vi "plain cycling.vi"() -> ()   [LabVIEW 2014]
doc: "This VI demonstrates the individual configuration of settings in I/W, W/I, and continuous operation modes.\n\nThis VI is not meant to be used with infusion-only models. \n\nNotes:\n(1) If continuous mode is selected, infuse volumes/rates will be used."
uses:
  <instrlib>/KD Scientific 2XX Series/KD Scientific 2XX Series.lvlib
panel:
  out "pressure mm Hg":dbl[](array[numeric])
  in  "Zero Error":dbl[](array[numeric])
  in  "Calibration factor":dbl[](array[numeric])
  out "Pressure mm Hg":dbl[](graph)
  out "Voltage from pressure transducer":dbl[](array[numeric])
  out "Data from Transducer":dynamicdata(graph) caption="Voltage from Transducer V"
  in  "stop (F)":bool
  in  "Number of Cycles":i32
  in  "Min Pressure":dbl
  in  "Max Pressure":dbl
  out "Units":string
  out "Delivered Volume":dbl
  in  "stop":bool
  out "Status":T1
  in  "Baud Rate (9600)":u32(ring)=9600 items=["300"=300, "1200"=1200, "2400"=2400, "4800"=4800, "9600"=9600]
  in  "Withdrawal Settings":T2={"Flow Rate (5)"=5.0, "Volume (10)"=10.0, "Volume Units (ml)"=enum."milliliters (ml)", "Rate Units (ml/min.)"=enum."milliliters per minute (ml/min.)"} {"Volume (10)" format="%#.3g"}
  in  "Diameter (8.75 mm)":dbl=8.75
  in  "Infusion Settings":T2={"Flow Rate (5)"=5.0, "Volume (10)"=10.0, "Volume Units (ml)"=enum."milliliters (ml)", "Rate Units (ml/min.)"=enum."milliliters per minute (ml/min.)"}
  in  "Address (0)":i32 format="%0.0f"
  in  "error in (no error)":errorcluster
  in  "VISA resource name":refnum<visa-resource-name>="COM1"
  # "RS-232 Settings"
  # "General Settings"
  # "Pump Status"
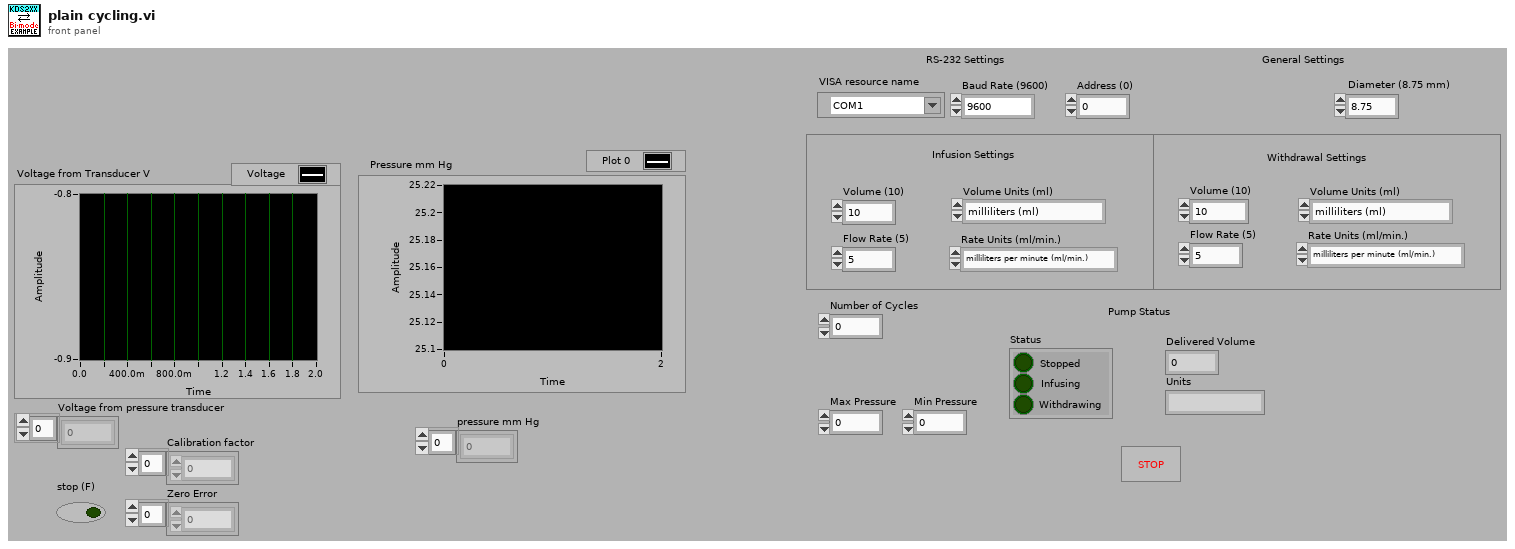
[diagram p1: front panel]
types:
  T1 = cluster{"Stopped":bool, "Infusing":bool, "Withdrawing":bool}
  T2 = cluster{"Flow Rate (5)":dbl, "Volume (10)":dbl, "Volume Units (ml)":enum16{"milliliters (ml)", "microliters (ul)"}, "Rate Units (ml/min.)":enum16{"milliliters per minute (ml/min.)", "milliliters per hour (ml/hr.)", "microliters per minute (ul/min.)", "microliters per hour (ul/hr.)"}}
  T3 = enum16{"milliliters per minute (ml/min.)", "milliliters per hour (ml/hr.)", "microliters per minute (ul/min.)", "microliters per hour (ul/hr.)"}
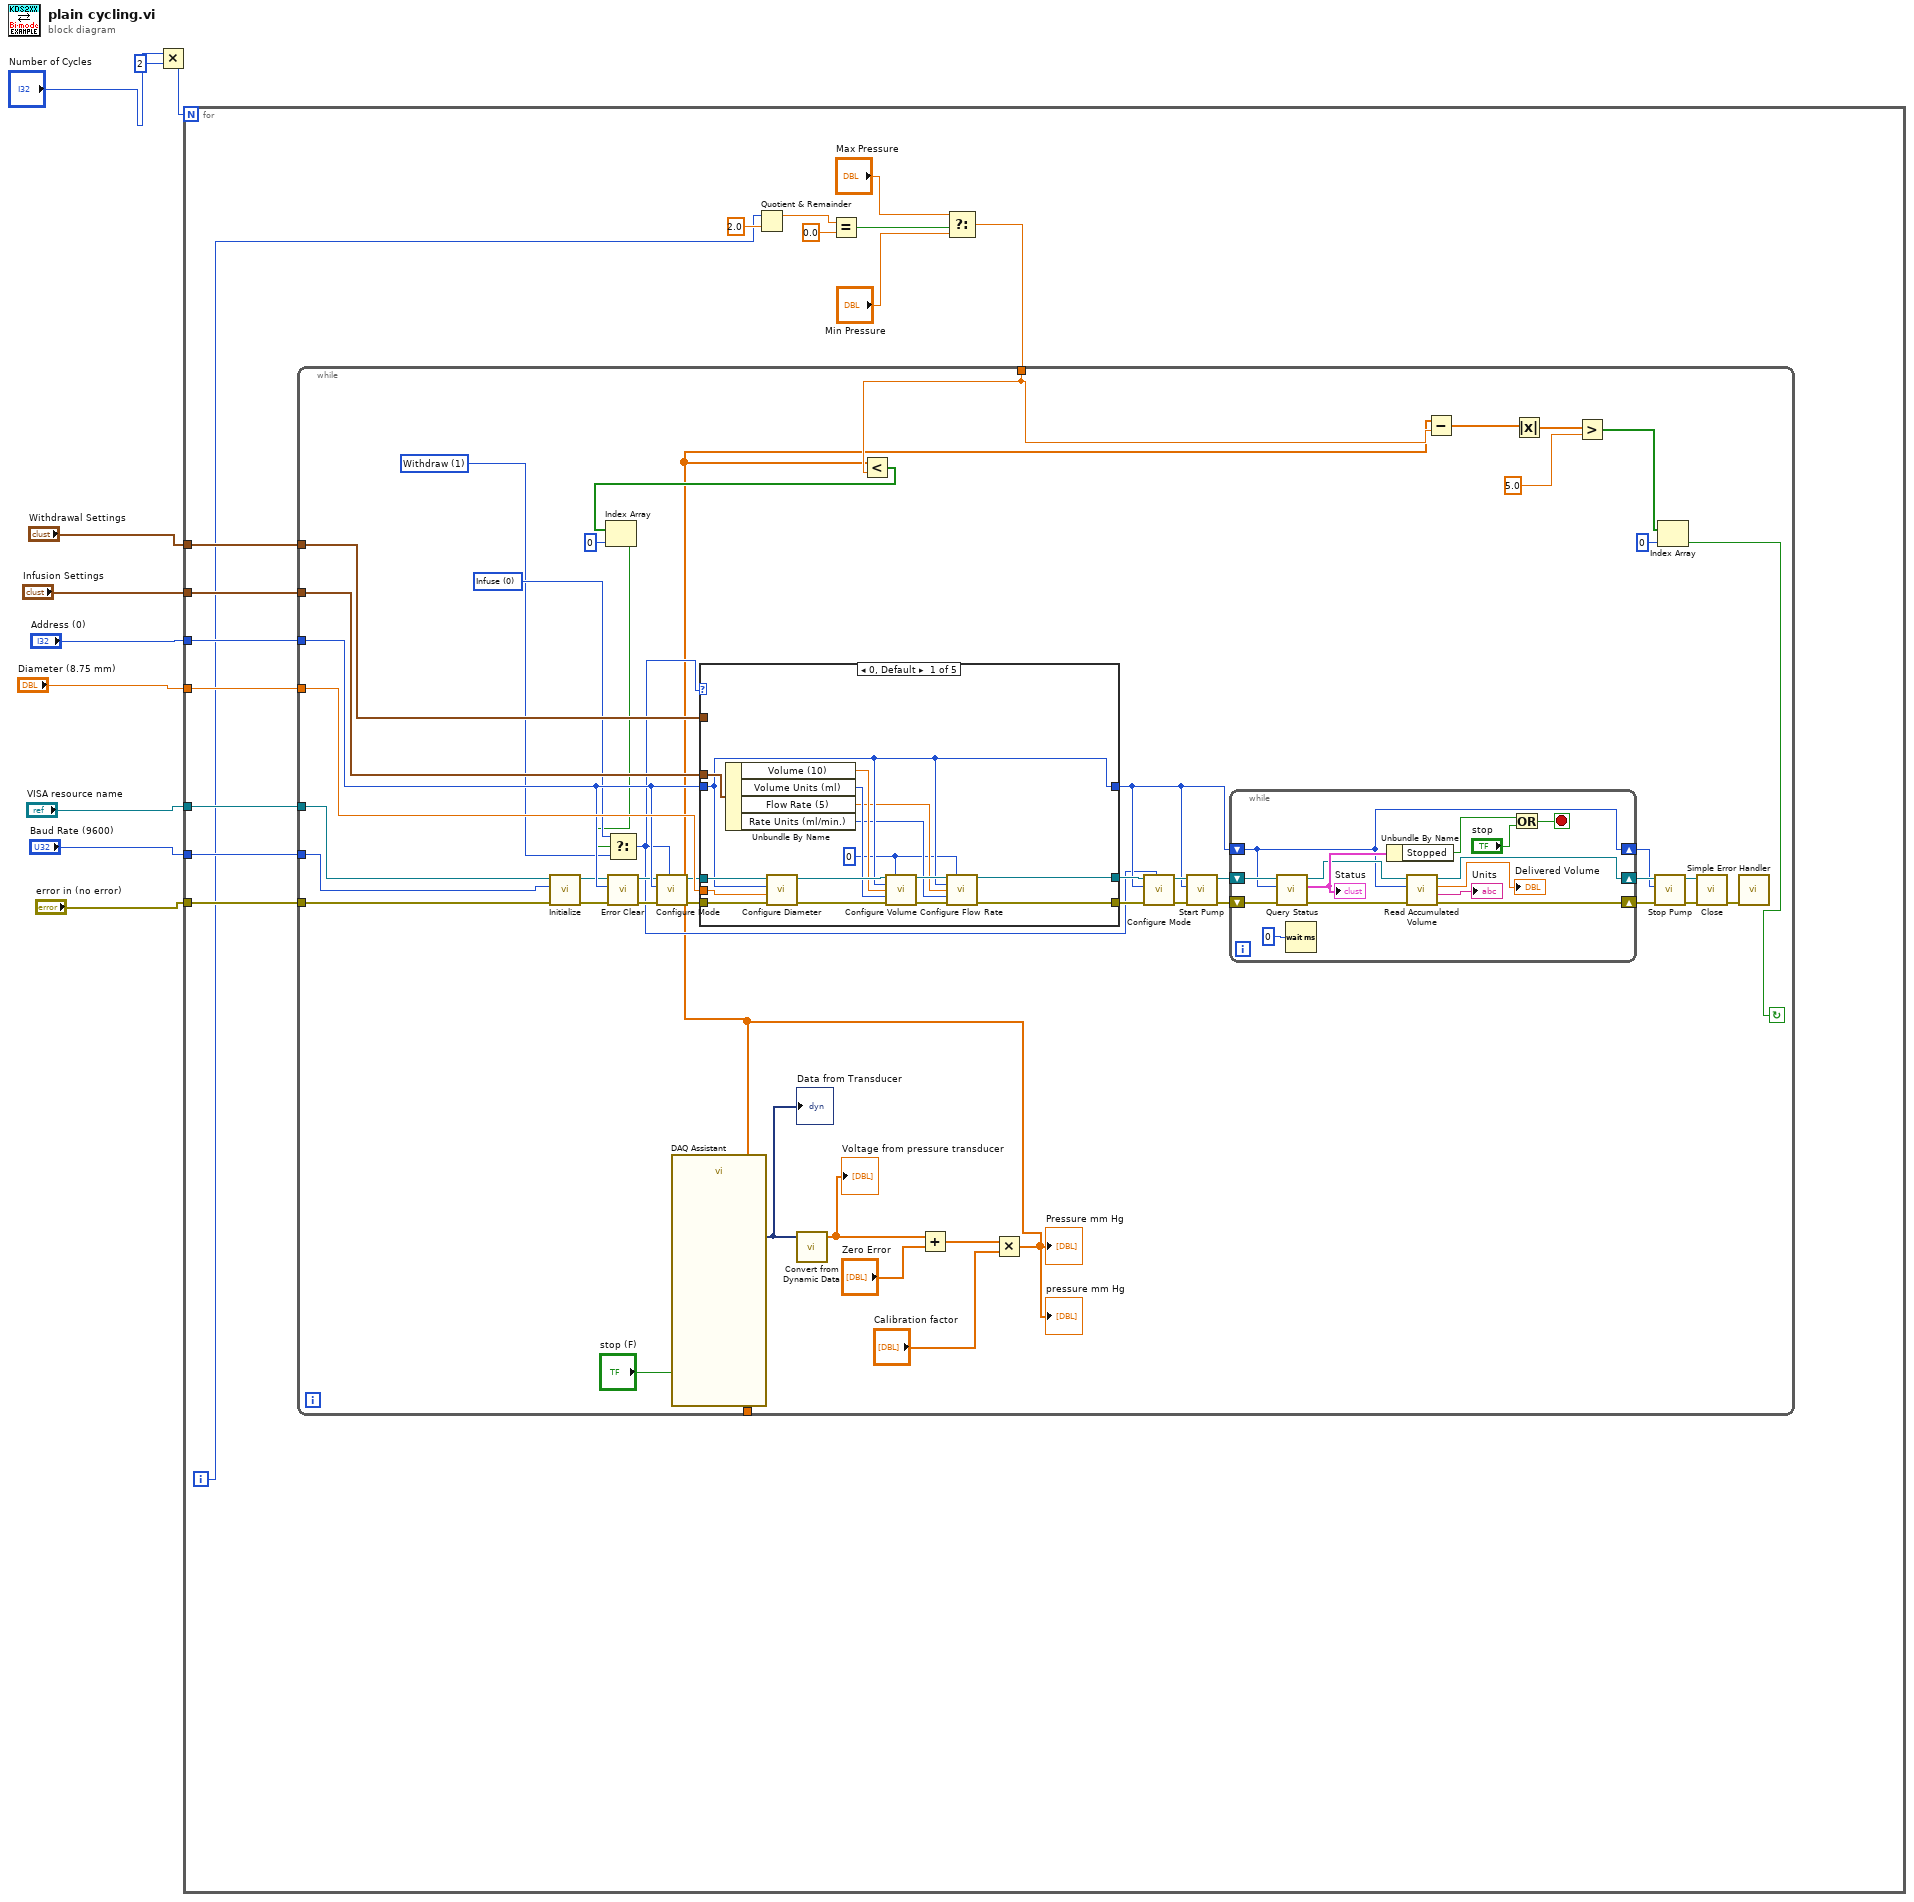
[diagram p0: block diagram]
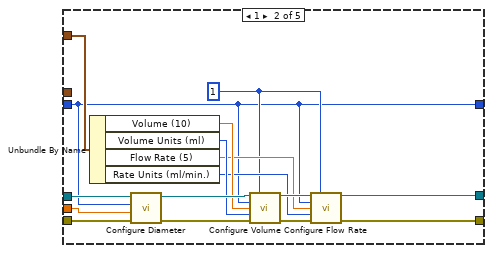
[diagram p2: hidden frame]
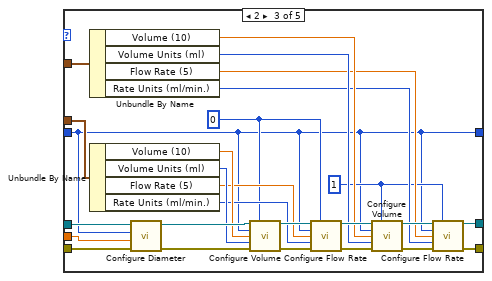
[diagram p3: hidden frame]
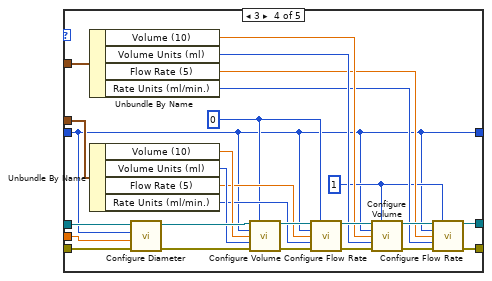
[diagram p4: hidden frame]
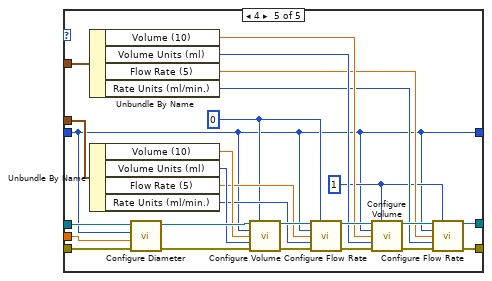
[diagram p5: hidden frame]
diagram:
  n1 = Multiply(x="Number of Cycles", y=2) -> (x*y=w1:i32)
  n2 = for {
    N: w1 -> [_]
    tunnel: "VISA resource name" -> [w25]
    tunnel: "error in (no error)" -> [w24]
    tunnel: "Infusion Settings" -> [w23]
    tunnel: "Withdrawal Settings" -> [w22]
    tunnel: "Diameter (8.75 mm)" -> [w21]
    tunnel: "Baud Rate (9600)" -> [w20]
    tunnel: "Address (0)" -> [w19]
    i -> [w17]
    n3 = Quotient & Remainder(x=w17, y=2.0) -> (x-y*floor(x/y)=w15:dbl)  [unwired: 1 out]
    n4 = Equal?(x=w15, y=0.0) -> (x = y?=w14:bool)
    n5 = Select(t="Max Pressure", s=w14, f="Min Pressure") -> (s? t:f=w11:dbl)
    n6 = while {
      tunnel: w25 -> [w71]
      tunnel: w24 -> [w70]
      tunnel: w23 -> [w69]
      tunnel: w22 -> [w68]
      tunnel: w21 -> [w67]
      tunnel: w20 -> [w66]
      tunnel: w19 -> [w65]
      tunnel: w11 -> [w42]
      tunnel: [w26] -> _
      stop <- w33 continue-if-true
      w44 = u16 1 items=["Withdraw"=1]
      w45 = u16 0 items=["Infuse"] ("Mode (infuse)")
      n7 = call <instrlib>:"Initialize.vi"("error in (no error)"=w70, "Baud Rate (9600)"=w66, "VISA resource name"=w71) -> ("error out"=w47:errorcluster, "VISA resource name out"=w46:refnum<visa-resource-name>)  [unwired: 7 in]
      n8 = call <instrlib>:"Error Clear.vi"("error in (no error)"=w47, "Address (0)"=w65, "VISA resource name"=w46) -> ("error out"=w48:errorcluster, "VISA resource name out"=w49:refnum<visa-resource-name>)  [unwired: 6 in, 1 out]
      n9 = call "DAQ Assistant"("stop (F)"="stop (F)") -> ("data"=w32:dynamicdata)  [unwired: 15 in, 3 out]
      "Data from Transducer" <- w32
      n10 = call "Convert from Dynamic Data"("Dynamic Data Type"=w32) -> ("Array"=w29:dbl[])  [unwired: 3 in]
      "Voltage from pressure transducer" <- w29
      n11 = Add(x=w29, y="Zero Error") -> (x+y=w31:dbl[])
      n12 = Multiply(x=w31, y="Calibration factor") -> (x*y=w26:dbl[])
      "Pressure mm Hg" <- w26
      "pressure mm Hg" <- w26
      n13 = Less?(x=w26, y=w42) -> (x < y?=w38:bool[])
      n14 = Index Array(array=w38, index=0) -> (element=w36:bool)
      n15 = Select(t=w45, s=w36, f=w44) -> (s? t:f=w43:u16)
      n16 = call <instrlib>:"Configure Mode.vi"("Mode (infuse)"=w43, "error in (no error)"=w48, "Address (0)"=w65, "VISA resource name"=w49) -> ("error out"=w51:errorcluster, "VISA resource name out"=w50:refnum<visa-resource-name>)  [unwired: 6 in]
      n17 = case shown="0, Default" w43 {
        tunnel: w69 -> [w81 _ w129 w155 w181]
        tunnel: w68 -> [_ w103 w128 w154 w180]
        tunnel: w50 -> [w87 w102 w127 w153 w179]
        tunnel: w51 -> [w86 w98 w126 w152 w178]
        tunnel: w67 -> [w80 w94 w109 w135 w161]
        tunnel: [w79 w88 w104 w130 w156] -> w52
        tunnel: w65 -> [w79 w88 w104 w130 w156]
        tunnel: [w74 w99 w106 w132 w158] -> w56
        tunnel: [w73 w95 w105 w131 w157] -> w55
        frame 0, Default {
          w72 = 0
          n18 = Unbundle By Name(w81) -> ("Volume (10)"=w78:dbl, "Volume Units (ml)"=w77:enum16{"milliliters (ml)", "microliters (ul)"}, "Flow Rate (5)"=w76:dbl, "Rate Units (ml/min.)"=w75:T3)
          n19 = call <instrlib>:"Configure Diameter.vi"("error in (no error)"=w86, "Diameter (8.75 mm)"=w80, "Address (0)"=w79, "VISA resource name"=w87) -> ("error out"=w84:errorcluster, "VISA resource name out"=w85:refnum<visa-resource-name>)  [unwired: 6 in]
          n20 = call <instrlib>:"Configure Volume.vi"("VISA resource name"=w85, "Mode (infuse)"=w72, "Address (0)"=w79, "Volume (100)"=w78, "Units (0: milliliters)"=w77, "error in (no error)"=w84) -> ("VISA resource name out"=w83:refnum<visa-resource-name>, "error out"=w82:errorcluster)  [unwired: 8 in]
          n21 = call <instrlib>:"Configure Flow Rate.vi"("VISA resource name"=w83, "Mode (infuse)"=w72, "Address (0)"=w79, "Flow Rate (5)"=w76, "Units (0: milliliters per minute)"=w75, "error in (no error)"=w82) -> ("VISA resource name out"=w74:refnum<visa-resource-name>, "error out"=w73:errorcluster)  [unwired: 8 in]
        }
        frame 1 {
          w89 = 1
          n22 = Unbundle By Name(w103) -> ("Volume (10)"=w93:dbl, "Volume Units (ml)"=w92:enum16{"milliliters (ml)", "microliters (ul)"}, "Flow Rate (5)"=w91:dbl, "Rate Units (ml/min.)"=w90:T3)
          n23 = call <instrlib>:"Configure Diameter.vi"("error in (no error)"=w98, "Diameter (8.75 mm)"=w94, "Address (0)"=w88, "VISA resource name"=w102) -> ("error out"=w97:errorcluster, "VISA resource name out"=w101:refnum<visa-resource-name>)  [unwired: 6 in]
          n24 = call <instrlib>:"Configure Volume.vi"("VISA resource name"=w101, "Mode (infuse)"=w89, "Address (0)"=w88, "Volume (100)"=w93, "Units (0: milliliters)"=w92, "error in (no error)"=w97) -> ("VISA resource name out"=w100:refnum<visa-resource-name>, "error out"=w96:errorcluster)  [unwired: 8 in]
          n25 = call <instrlib>:"Configure Flow Rate.vi"("VISA resource name"=w100, "Mode (infuse)"=w89, "Address (0)"=w88, "Flow Rate (5)"=w91, "Units (0: milliliters per minute)"=w90, "error in (no error)"=w96) -> ("VISA resource name out"=w99:refnum<visa-resource-name>, "error out"=w95:errorcluster)  [unwired: 8 in]
        }
        frame 2 {
          w107 = 1
          w108 = 0
          n26 = Unbundle By Name(w128) -> ("Volume (10)"=w113:dbl, "Volume Units (ml)"=w112:enum16{"milliliters (ml)", "microliters (ul)"}, "Flow Rate (5)"=w111:dbl, "Rate Units (ml/min.)"=w110:T3)
          n27 = Unbundle By Name(w129) -> ("Volume (10)"=w117:dbl, "Volume Units (ml)"=w116:enum16{"milliliters (ml)", "microliters (ul)"}, "Flow Rate (5)"=w115:dbl, "Rate Units (ml/min.)"=w114:T3)
          n28 = call <instrlib>:"Configure Diameter.vi"("error in (no error)"=w126, "Diameter (8.75 mm)"=w109, "Address (0)"=w104, "VISA resource name"=w127) -> ("error out"=w121:errorcluster, "VISA resource name out"=w125:refnum<visa-resource-name>)  [unwired: 6 in]
          n29 = call <instrlib>:"Configure Volume.vi"("VISA resource name"=w125, "Mode (infuse)"=w108, "Address (0)"=w104, "Volume (100)"=w117, "Units (0: milliliters)"=w116, "error in (no error)"=w121) -> ("VISA resource name out"=w124:refnum<visa-resource-name>, "error out"=w120:errorcluster)  [unwired: 8 in]
          n30 = call <instrlib>:"Configure Flow Rate.vi"("VISA resource name"=w124, "Mode (infuse)"=w108, "Address (0)"=w104, "Flow Rate (5)"=w115, "Units (0: milliliters per minute)"=w114, "error in (no error)"=w120) -> ("VISA resource name out"=w123:refnum<visa-resource-name>, "error out"=w119:errorcluster)  [unwired: 8 in]
          n31 = call <instrlib>:"Configure Volume.vi"("VISA resource name"=w123, "Mode (infuse)"=w107, "Address (0)"=w104, "Volume (100)"=w113, "Units (0: milliliters)"=w112, "error in (no error)"=w119) -> ("VISA resource name out"=w122:refnum<visa-resource-name>, "error out"=w118:errorcluster)  [unwired: 8 in]
          n32 = call <instrlib>:"Configure Flow Rate.vi"("VISA resource name"=w122, "Mode (infuse)"=w107, "Address (0)"=w104, "Flow Rate (5)"=w111, "Units (0: milliliters per minute)"=w110, "error in (no error)"=w118) -> ("VISA resource name out"=w106:refnum<visa-resource-name>, "error out"=w105:errorcluster)  [unwired: 8 in]
        }
        frame 3 {
          w133 = 1
          w134 = 0
          n33 = Unbundle By Name(w154) -> ("Volume (10)"=w139:dbl, "Volume Units (ml)"=w138:enum16{"milliliters (ml)", "microliters (ul)"}, "Flow Rate (5)"=w137:dbl, "Rate Units (ml/min.)"=w136:T3)
          n34 = Unbundle By Name(w155) -> ("Volume (10)"=w143:dbl, "Volume Units (ml)"=w142:enum16{"milliliters (ml)", "microliters (ul)"}, "Flow Rate (5)"=w141:dbl, "Rate Units (ml/min.)"=w140:T3)
          n35 = call <instrlib>:"Configure Diameter.vi"("error in (no error)"=w152, "Diameter (8.75 mm)"=w135, "Address (0)"=w130, "VISA resource name"=w153) -> ("error out"=w147:errorcluster, "VISA resource name out"=w151:refnum<visa-resource-name>)  [unwired: 6 in]
          n36 = call <instrlib>:"Configure Volume.vi"("VISA resource name"=w151, "Mode (infuse)"=w134, "Address (0)"=w130, "Volume (100)"=w143, "Units (0: milliliters)"=w142, "error in (no error)"=w147) -> ("VISA resource name out"=w150:refnum<visa-resource-name>, "error out"=w146:errorcluster)  [unwired: 8 in]
          n37 = call <instrlib>:"Configure Flow Rate.vi"("VISA resource name"=w150, "Mode (infuse)"=w134, "Address (0)"=w130, "Flow Rate (5)"=w141, "Units (0: milliliters per minute)"=w140, "error in (no error)"=w146) -> ("VISA resource name out"=w149:refnum<visa-resource-name>, "error out"=w145:errorcluster)  [unwired: 8 in]
          n38 = call <instrlib>:"Configure Volume.vi"("VISA resource name"=w149, "Mode (infuse)"=w133, "Address (0)"=w130, "Volume (100)"=w139, "Units (0: milliliters)"=w138, "error in (no error)"=w145) -> ("VISA resource name out"=w148:refnum<visa-resource-name>, "error out"=w144:errorcluster)  [unwired: 8 in]
          n39 = call <instrlib>:"Configure Flow Rate.vi"("VISA resource name"=w148, "Mode (infuse)"=w133, "Address (0)"=w130, "Flow Rate (5)"=w137, "Units (0: milliliters per minute)"=w136, "error in (no error)"=w144) -> ("VISA resource name out"=w132:refnum<visa-resource-name>, "error out"=w131:errorcluster)  [unwired: 8 in]
        }
        frame 4 {
          w159 = 1
          w160 = 0
          n40 = Unbundle By Name(w180) -> ("Volume (10)"=w165:dbl, "Volume Units (ml)"=w164:enum16{"milliliters (ml)", "microliters (ul)"}, "Flow Rate (5)"=w163:dbl, "Rate Units (ml/min.)"=w162:T3)
          n41 = Unbundle By Name(w181) -> ("Volume (10)"=w169:dbl, "Volume Units (ml)"=w168:enum16{"milliliters (ml)", "microliters (ul)"}, "Flow Rate (5)"=w167:dbl, "Rate Units (ml/min.)"=w166:T3)
          n42 = call <instrlib>:"Configure Diameter.vi"("error in (no error)"=w178, "Diameter (8.75 mm)"=w161, "Address (0)"=w156, "VISA resource name"=w179) -> ("error out"=w173:errorcluster, "VISA resource name out"=w177:refnum<visa-resource-name>)  [unwired: 6 in]
          n43 = call <instrlib>:"Configure Volume.vi"("VISA resource name"=w177, "Mode (infuse)"=w160, "Address (0)"=w156, "Volume (100)"=w169, "Units (0: milliliters)"=w168, "error in (no error)"=w173) -> ("VISA resource name out"=w176:refnum<visa-resource-name>, "error out"=w172:errorcluster)  [unwired: 8 in]
          n44 = call <instrlib>:"Configure Flow Rate.vi"("VISA resource name"=w176, "Mode (infuse)"=w160, "Address (0)"=w156, "Flow Rate (5)"=w167, "Units (0: milliliters per minute)"=w166, "error in (no error)"=w172) -> ("VISA resource name out"=w175:refnum<visa-resource-name>, "error out"=w171:errorcluster)  [unwired: 8 in]
          n45 = call <instrlib>:"Configure Volume.vi"("VISA resource name"=w175, "Mode (infuse)"=w159, "Address (0)"=w156, "Volume (100)"=w165, "Units (0: milliliters)"=w164, "error in (no error)"=w171) -> ("VISA resource name out"=w174:refnum<visa-resource-name>, "error out"=w170:errorcluster)  [unwired: 8 in]
          n46 = call <instrlib>:"Configure Flow Rate.vi"("VISA resource name"=w174, "Mode (infuse)"=w159, "Address (0)"=w156, "Flow Rate (5)"=w163, "Units (0: milliliters per minute)"=w162, "error in (no error)"=w170) -> ("VISA resource name out"=w158:refnum<visa-resource-name>, "error out"=w157:errorcluster)  [unwired: 8 in]
        }
      }
      n47 = call <instrlib>:"Configure Mode.vi"("Mode (infuse)"=w43, "error in (no error)"=w55, "Address (0)"=w52, "VISA resource name"=w56) -> ("error out"=w53:errorcluster, "VISA resource name out"=w54:refnum<visa-resource-name>)  [unwired: 6 in]
      n48 = call <instrlib>:"Start Pump.vi"("error in (no error)"=w53, "Address (0)"=w52, "VISA resource name"=w54) -> ("error out"=w63:errorcluster, "VISA resource name out"=w64:refnum<visa-resource-name>)  [unwired: 7 in]
      n49 = while {
        shift-right: [w184] -> w60
        shift-left: w52 -> [w184]
        shift-right: [w186] -> w62
        shift-left: w64 -> [w192]
        shift-right: [w185] -> w61
        shift-left: w63 -> [w193]
        stop <- w190 stop-if-true
        n50 = call <instrlib>:"Query Status.vi"("error in (no error)"=w193, "Address (0)"=w184, "VISA resource name"=w192) -> ("error out"=w195:errorcluster, "Status"=w191:T1, "VISA resource name out"=w187:refnum<visa-resource-name>)  [unwired: 6 in]
        "Status" <- w191
        n51 = Wait (ms)(milliseconds to wait=u32 0) -> ()  [unwired: 1 out]
        n52 = Unbundle By Name(w191) -> ("Stopped"=w189:bool)
        n53 = call <instrlib>:"Read Accumulated Volume.vi"("error in (no error)"=w195, "Address (0)"=w184, "VISA resource name"=w187) -> ("error out"=w185:errorcluster, "Units"=→"Units":string, "Delivered Volume"=→"Delivered Volume":dbl, "VISA resource name out"=w186:refnum<visa-resource-name>)  [unwired: 5 in]
        n54 = Or(x=w189, y="stop") -> (x .or. y?=w190:bool)
      }
      n55 = Subtract(x=w26, y=w42) -> (x-y=w41:dbl[])
      n56 = Absolute Value(x=w41) -> (abs(x)=w40:dbl[])
      n57 = Greater?(x=w40, y=5.0) -> (0:w35:bool[])
      n58 = call <instrlib>:"Stop Pump.vi"("error in (no error)"=w61, "Address (0)"=w60, "VISA resource name"=w62) -> ("error out"=w58:errorcluster, "VISA resource name out"=w57:refnum<visa-resource-name>)  [unwired: 7 in]
      n59 = Index Array(array=w35, index=0) -> (element=w33:bool)
      n60 = call <instrlib>:"Close.vi"("error in (no error)"=w58, "VISA resource name"=w57) -> ("error out"=w59:errorcluster)  [unwired: 9 in]
      n61 = call <vilib>:"Simple Error Handler.vi"("error in (no error)"=w59) -> ()  [unwired: 4 in, 5 out]
    }
  }
